vi "HandleDeletedWindowDVR.vi"(7 "Window To Handle In":map{refnum<class "Window.lvclass">, i64}(c390), 8 "error in (no error)":errorcluster, 10 "Window":refnum<class "Window.lvclass">, 11 "Replace Action In":T1=enum."Add or Modify Entry") -> (0 "error out":errorcluster, 3 "Replace Action Out":T1, 5 "Window To Handle Out":map{refnum<class "Window.lvclass">, i64}(c390))   [LabVIEW 2020, in "GLF.lvlib" / "Engine.lvclass"]
uses:
  Engine.lvclass
  Window/Window.lvclass
  Engine.lvclass/Engine.ctl
  <vilib>/Utility/miscctls.llb/LVMapReplaceAction.ctl
  <vilib>/Saukko/LV SDL3/Sources/SDL3/Video/Video.lvlib
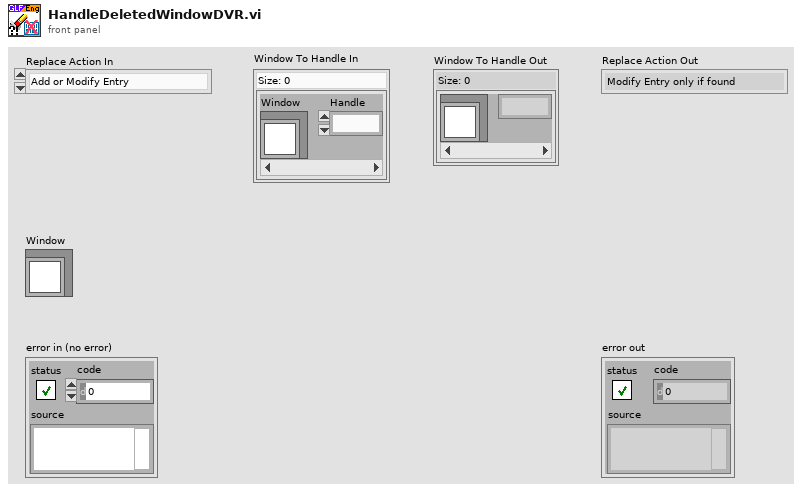
[diagram p1: front panel]
types:
  T1 = typedef "LVMapReplaceAction.ctl" = enum32{"Modify Entry only if found", "Add or Modify Entry", "Delete Entry"}
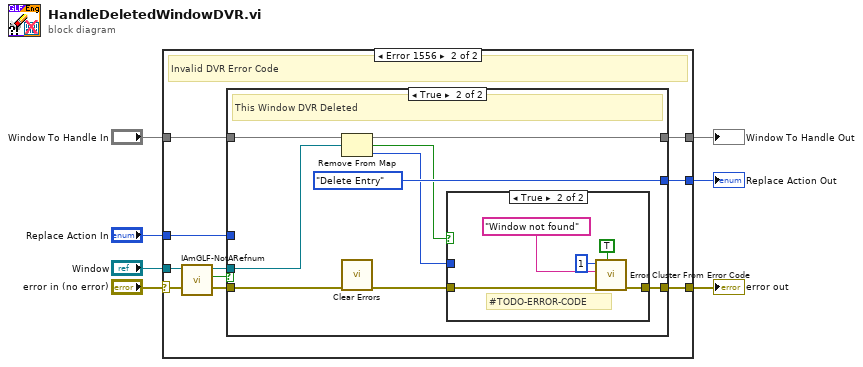
[diagram p0: block diagram]
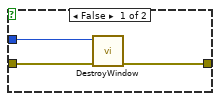
[diagram p4: hidden frame]
diagram:
  n1 = case shown="Error 1556" "error in (no error)" {
    selector: "error in (no error)" -> [w10 w19]
    tunnel: [w10 w17] -> w6
    tunnel: "Window" -> [_ w18]
    tunnel: "Replace Action In" -> [w9 w15]
    tunnel: [w9 w14] -> w3
    tunnel: "Window To Handle In" -> [w8 w12]
    tunnel: [w8 w13] -> w1
    frame No Error {
      # "Do nothing"
      # "Other"
    }
    frame Error {
      # "Invalid DVR Error Code"
      n2 = call-dynamic "IAmGLF-NotARefnum.vi"("Window in"=w18) -> ("Not A Valid Refnum?"=w16:bool, "Window out"=w11:refnum<class "Window.lvclass">)  [unwired: 9 in]
      n3 = case shown="True" w16 {
        tunnel: w19 -> [w22 w31]
        tunnel: [w22 w25] -> w17
        tunnel: w15 -> [w21 _]
        tunnel: [w21 LVMapReplaceAction."Delete Entry" ("Replace Action In")] -> w14
        tunnel: [w20 w26] -> w13
        tunnel: w12 -> [w20 w28]
        tunnel: w11 -> [_ w27]
        frame False {
          # "Other DVR Error"
        }
        frame True {
          # "This Window DVR Deleted"
          n4 = Remove From Map(10:w27, 11:w28) -> (1:w24:i64, 2:w23:bool, 3:w26:map{refnum<class "Window.lvclass">, i64})
          n5 = call <vilib>:"Clear Errors.vi"("error in (no error)"=w31) -> ("error out"=w30:errorcluster)  [unwired: 5 in, 1 out]
          n6 = case shown="True" w23 {
            tunnel: w30 -> [w34 w39]
            tunnel: [w33 w38] -> w25
            tunnel: w24 -> [w32 _]
            frame False {
              n7 = call <vilib>:"DestroyWindow.vi"("No Error"=w34, "Window [SDL_Window*]"=w32) -> ("Error Out"=w33:errorcluster)  [unwired: 9 in]
            }
            frame True {
              # "#TODO-ERROR-CODE"
              n8 = call <vilib>:"Error Cluster From Error Code.vi"("show call chain? (False)"=TRUE, "error in (no error)"=w39, "error message (\"\")"="Window not found" ("error message (\"\")"), "error code (0)"=1) -> ("error out"=w38:errorcluster)  [unwired: 5 in]
            }
          }
        }
      }
    }
  }
  "error out" <- w6
  "Replace Action Out" <- w3
  "Window To Handle Out" <- w1
